vi "Set Variant.vi"(8 "error in (no error)":errorcluster, 10 "Variant":variant, 11 "Message in":refnum<class "Raw Message.lvclass">) -> (0 "error out":errorcluster, 3 "Message out":refnum<class "Raw Message.lvclass">)   [LabVIEW 2020, in "Protobuf RAW.lvlib" / "Raw Message.lvclass"]
uses:
  Raw Message.lvclass
  Raw Message.lvclass/Raw Message.ctl
  Tag/Basic Type.lvclass
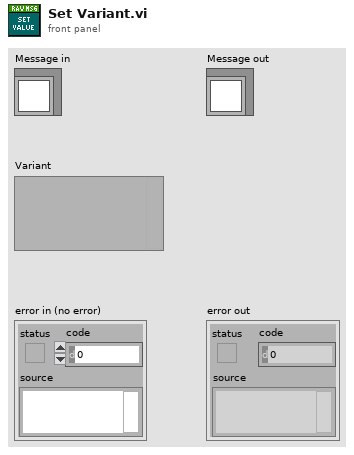
[diagram p1: front panel]
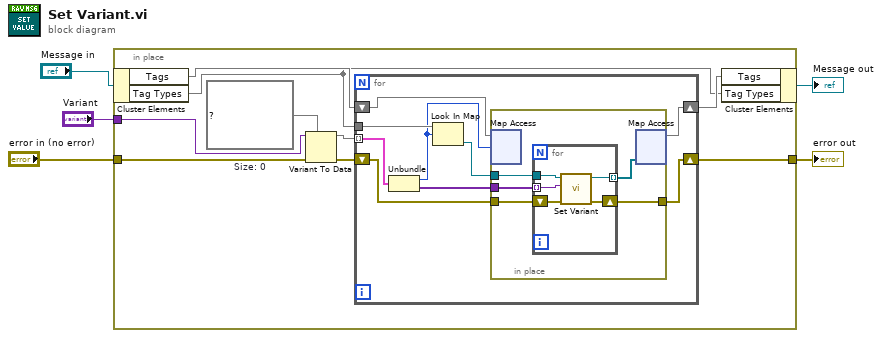
[diagram p0: block diagram]
diagram:
  n1 = in-place {
    in-place-border: "error in (no error)" -> [w14]
    in-place-border: "Variant" -> [w13]
    in-place-border: [w7] -> w1
    w10 = map{u32, variant[]} {}  # Size: 0
    n2 = in-place-cluster #1("Message in") -> ("Tags"=w8:map{u32, refnum<class "Basic Type.lvclass">[]}, "Tag Types"=w6:map{u32, refnum<class "Basic Type.lvclass">})
    n3 = Variant To Data(error in=w14, type=w10, Variant=w13) -> (data=w11:map{u32, variant[]}, error out=w12:errorcluster)
    n4 = for {
      tunnel: w11 -> [w23] mode=indexing
      shift-right: [w19] -> w7
      shift-left: w12 -> [w20]
      shift-right: [w21] -> w9
      shift-left: w8 -> [w22]
      tunnel: w6 -> [w17]
      n5 = Unbundle(w23) -> ("ID"=w16:u32, "Array"=w18:variant[])
      n6 = Look In Map(map=w17, key=w16) -> (value=w15:refnum<class "Basic Type.lvclass">)  [unwired: 1 in, 1 out]
      n7 = in-place {
        in-place-border: w20 -> [w27]
        in-place-border: [w26] -> w19
        in-place-border: w18 -> [w25]
        in-place-border: w15 -> [w24]
        n8 = in-place-map #2(w22, w16) -> ()  [unwired: 1 in, 2 out]
        n9 = for {
          tunnel: [w33] -> w28 mode=indexing
          shift-right: [w31] -> w26
          shift-left: w27 -> [w32]
          tunnel: w25 -> [w30] mode=indexing
          tunnel: w24 -> [w29]
          n10 = call-dynamic "Set Variant.vi"("error in (no error)"=w32, "Variant"=w30, "Type Serializer in"=w29) -> ("error out"=w31:errorcluster, "Type Serializer out"=w33:refnum<class "Basic Type.lvclass">)  [unwired: 7 in]
        }
        n11 = in-place-map #2(w28) -> (w21:map{u32, refnum<class "Basic Type.lvclass">[]})  [unwired: 1 in, 2 out]
      }
    }
    n12 = in-place-cluster #1("Tags"=w9, "Tag Types"=w6) -> (→"Message out":refnum<class "Raw Message.lvclass">)
  }
  "error out" <- w1
